vi "Write Size.vi"(8 "error in (no error)":errorcluster, 10 "Size":i32, 11 "Splitter in":refnum<class "Splitter.lvclass">) -> (0 "error out":errorcluster, 3 "Splitter out":refnum<class "Splitter.lvclass">)   [LabVIEW 2019, in "Splitter.lvclass"]
uses:
  <resource>/dialog/QuickDrop/plugins/PaneRelief/Classes/Splitter/Splitter.lvclass
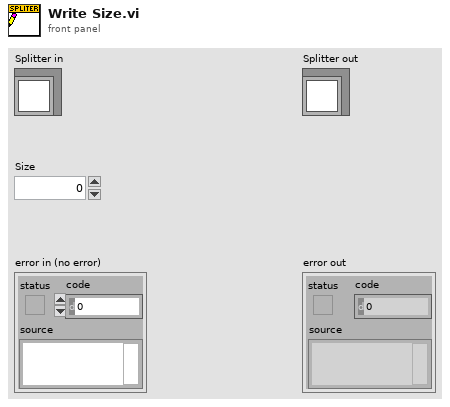
[diagram p1: front panel]
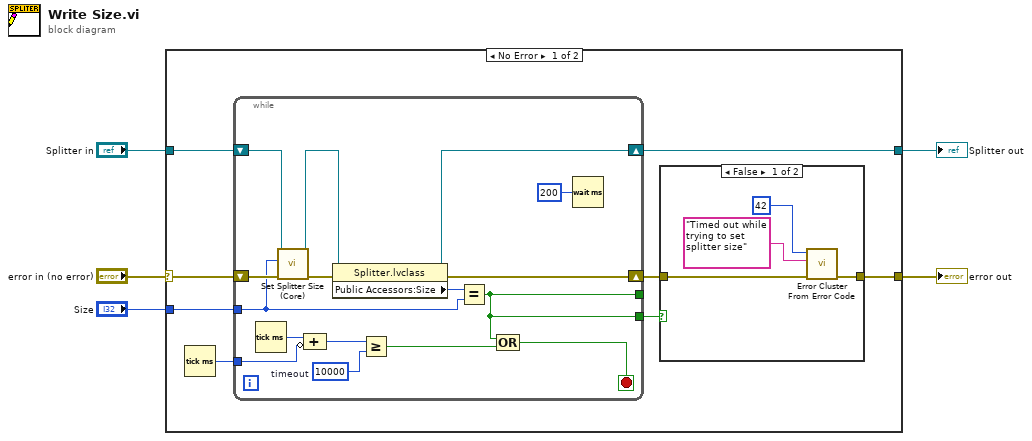
[diagram p0: block diagram]
diagram:
  n1 = case shown="No Error" "error in (no error)" {
    selector: "error in (no error)" -> [w6 w35]
    tunnel: [w7 w35] -> w4
    tunnel: "Size" -> [w13 _]
    tunnel: "Splitter in" -> [w12 w36]
    tunnel: [w11 w36] -> w1
    frame No Error {
      n2 = Tick Count (ms)() -> (millisecond timer value=w10:u32)
      n3 = while {
        tunnel: w13 -> [w23]
        shift-right: [w14] -> w9
        shift-left: w6 -> [w29]
        shift-right: [w25] -> w11
        shift-left: w12 -> [w27]
        tunnel: w10 -> [w20]
        tunnel: [w16] -> _
        tunnel: [w16] -> w8
        stop <- w22 stop-if-true
        w18 = u32 10000  # timeout
        n4 = Tick Count (ms)() -> (millisecond timer value=w21:u32)
        n5 = call <resource>:"Set Splitter Size (Core).vi"("error in (no error)"=w29, "Size"=w23, "Splitter in"=w27) -> ("error out"=w28:errorcluster, "Splitter out"=w26:refnum<class "Splitter.lvclass">)  [unwired: 7 in]
        n6 = Compound Arithmetic op=ADD(w21, invert w20) -> (w19:u32)
        n7 = property class="Splitter.lvclass"(reference=w26, error in=w28) -> (reference out=w25:refnum<class "Splitter.lvclass">, error out=w14:errorcluster, "Public Accessors:Size"=w24:i32)
        n8 = Greater Or Equal?(x=w19, y=w18) -> (x >= y?=w17:bool)
        n9 = Equal?(x=w24, y=w23) -> (x = y?=w16:bool)
        n10 = Compound Arithmetic op=OR(w16, w17) -> (w22:bool)
        n11 = Wait (ms)(milliseconds to wait=u32 200) -> ()  [unwired: 1 out]
      }
      n12 = case shown="False" w8 {
        tunnel: w9 -> [w33 w34]
        tunnel: [w32 w34] -> w7
        frame False {
          n13 = call <vilib>:"Error Cluster From Error Code.vi"("error in (no error)"=w33, "error message (\"\")"="Timed out while trying to set splitter size", "error code (0)"=42) -> ("error out"=w32:errorcluster)  [unwired: 6 in]
        }
        frame True {
        }
      }
    }
    frame Error {
    }
  }
  "error out" <- w4
  "Splitter out" <- w1
